vi "Register for Panel Events.vi"(8 "error in (no error)":errorcluster, 9 "Controls to Exclude":refnum<vi>[](array[refnum]), 10 "VI Refnum (Calling VI)":refnum<vi>, 11 "AbstractAutoRegistration In":refnum<class "AutoRegistration.lvclass">) -> (0 "error out":errorcluster, 1 "Stop! Event":refnum<user-event>, 2 "Auto-Event Registration Refnum":T1, 3 "AbstractAutoRegistration out":refnum<class "AutoRegistration.lvclass">)   [LabVIEW 2019, in "AutoRegistration.lvlib" / "AutoRegistration.lvclass"]
doc: "<License>\nCopyright © 2020 Tymphany, LLC | All rights reserved\nwww.Tymphany.com\nHuijun <Huijun.Guo@Tymphany.com>\n</License>"
uses:
  <vilib>/gpm_packages/@cs/mva-viewable/Source/ActorEvents/AutoRegistration/AutoRegistration.lvclass
  <vilib>/gpm_packages/@cs/mva-viewable/Source/ActorEvents/AutoRegistration/Auto-Event Registration Refnum.ctl
  <vilib>/gpm_packages/@cs/mva-viewable/Source/ActorEvents/AutoRegistration/Read Refnum Groups.vi
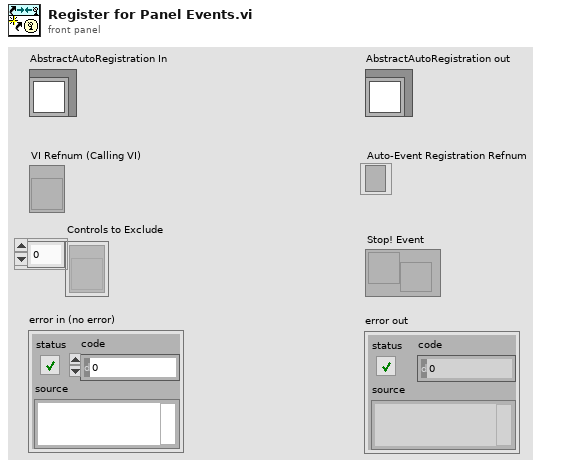
[diagram p1: front panel]
types:
  T1 = typedef "AutoRegistration.lvlib/AutoRegistration.lvclass/Auto-Event Registration Refnum.ctl" = refnum<event-registration>
  T2 = typedef "AutoRegistration.lvlib/AutoRegistration.lvclass/Registration References.ctl" = cluster{"Latching Boolean":refnum<vi>[], "Switching Boolean":refnum<vi>[], "Not Boolean":refnum<vi>[]}
  T3 = enum32{"Invalid", "Standard", "Closed", "Hidden", "Minimized", "Maximized"}
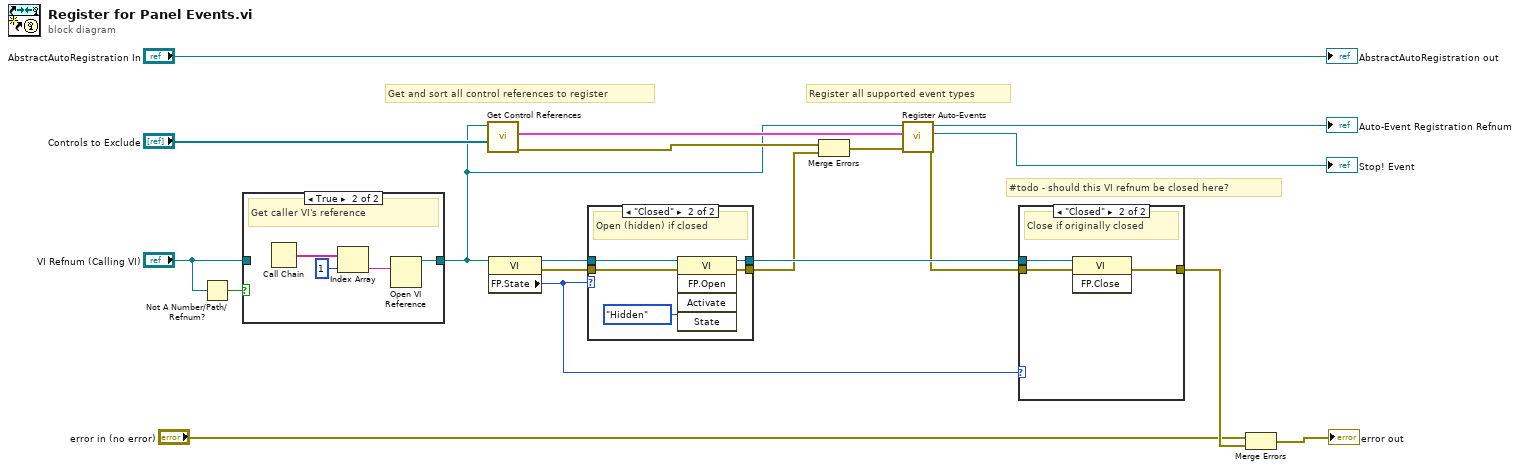
[diagram p0: block diagram]
diagram:
  # "#todo - should this VI refnum be closed here?"
  # "Register all supported event types"
  # "Get and sort all control references to register"
  n1 = Not A Number/Path/Refnum?(number/path/refnum="VI Refnum (Calling VI)") -> (NaN/Path/Refnum?=w12:bool)
  n2 = case shown="True" w12 {
    tunnel: [w20 w21] -> w5
    tunnel: "VI Refnum (Calling VI)" -> [w20 _]
    frame False {
      # "Reference wired to input"
    }
    frame True {
      # "Get caller VI's reference"
      n3 = Call Chain() -> (call chain=w24:string[])
      n4 = Index Array(array=w24, index=1) -> (element=w22:string)
      n5 = Open VI Reference(vi path=w22) -> (vi reference=w21:refnum<vi>)  [unwired: 5 in, 1 out]
    }
  }
  n6 = call <vilib>:"Get Control References.vi"("Controls to Exclude"="Controls to Exclude", "VI Refnum"=w5) -> ("error out"=w11:errorcluster, "Controls"=w9:T2)  [unwired: 8 in]
  n7 = property on="Property Node" class="VI"(reference=w5) -> (reference out=w3:refnum<vi>, error out=w2:errorcluster, "FP.State"=w18:T3)  [unwired: 1 in]
  n8 = case shown="\"Closed\"" w18 {
    tunnel: w3 -> [w26 w30]
    tunnel: [w25 w29] -> w15
    tunnel: [w26 w28] -> w19
    tunnel: w2 -> [w25 w27]
    frame Default {
    }
    frame "Closed" {
      # "Open (hidden) if closed"
      n9 = invoke on="Invoke Node" class="VI" method="FP.Open"(reference=w30, error in=w27, "State"=T3."Hidden") -> (reference out=w28:refnum<vi>, error out=w29:errorcluster)  [unwired: 2 in, 3 out]
    }
  }
  n10 = Merge Errors(w11, w15) -> (w8:errorcluster)
  n11 = call <vilib>:"Register Auto-Events.vi"("error in (no error)"=w8, "Controls"=w9, "VI"=w5) -> ("error out"=w6:errorcluster, "Stop!"=→"Stop! Event":refnum<user-event>, "Auto-Event Registration Refnum"=→"Auto-Event Registration Refnum":T1)  [unwired: 6 in]
  n12 = case shown="\"Closed\"" w18 {
    tunnel: w19 -> [_ w35]
    tunnel: [w32 w34] -> w17
    tunnel: w6 -> [w32 w33]
    frame Default {
    }
    frame "Closed" {
      # "Close if originally closed"
      n13 = invoke on="Invoke Node" class="VI" method="FP.Close"(reference=w35, error in=w33) -> (error out=w34:errorcluster)  [unwired: 1 in, 2 out]
    }
  }
  n14 = Merge Errors("error in (no error)", w17) -> (→"error out":errorcluster)
  "AbstractAutoRegistration out" <- "AbstractAutoRegistration In"
